vi "Test DAQmx With Queues.vi"() -> ()   [LabVIEW 2019, in "DAQmx.lvclass"]
uses:
  DAQmx.lvclass
  typedefs/DAQ.Configuration--Cluster.ctl
  typedefs/DAQ.Config.Timing--Cluster.ctl
  typedefs/DAQ.Config.Timing.Sampling--Cluster.ctl
  typedefs/DAQ.Config.Timing.Fs Mode--enum.ctl
  typedefs/DAQ.Config.AO--Cluster--Array.ctl
  typedefs/DAQ.Config.AO--Cluster.ctl
  typedefs/DAQ.Config.AO.Range--enum.ctl
  typedefs/DAQ.Config.Device Type--enum.ctl
  typedefs/DAQ.Config.AI--Cluster--Array.ctl
  typedefs/DAQ.Config.AI--Cluster.ctl
  typedefs/DAQ.Config.AI.Coupling--enum.ctl
  typedefs/DAQ.Config.AI.Range--enum.ctl
  typedefs/DAQ.Calibration--Cluster--Array.ctl
  typedefs/DAQ.Calibration--Cluster.ctl
  DAQmx.lvclass/DAQmx.ctl
panel:
  out "Waveform Chart":i32(graph)
  out "Generator create":i32
  out "Generator 'timeout'":i32
  out "DAQ 'timeout'":i32
  out "Generator":i32
  out "DAQ":i32
  out "Waveform Graph":waveform(dbl)[](graph)
  in  "stop":bool
  in  "Configuration":T1={"Timing"={"Sampling"={"Fs"=52000.0, "#s"=5000}, "sample mode"=10123, "FsMode"=enum."Manual", "Fs Multiplier"=1.0, "Refresh Rate (Hz)"=10.0, "Decimation.PreDSP"=1, "Decimation.PostDSP"=1, "Fs.Output"=204789.0}, "AO"=[{"Channels"="PXI1Slot3/ao0", "Range"=enum."±1.0", "output terminal configuration"=-1, "Type"=enum."None"}, {"Channels"="PXI1Slot3/ao1", "Range"=enum."±1.0", "output terminal configuration"=-1, "Type"=enum."None"}, {"Channels"="PXI1Slot5/ao0", "Range"=enum."±1.0", "output terminal configuration"=-1, "Type"=enum."None"}, {"Channels"="PXI1Slot5/ao1", "Range"=enum."±1.0", "output terminal configuration"=-1, "Type"=enum."None"}], "AI"=[{"Channels"="PXI1Slot3/ai0", "Coupling"=10050, "Range"=enum."±0.316", "input terminal configuration"=-1, "Type"=enum."None"}, {"Channels"="PXI1Slot3/ai1", "Coupling"=10050, "Range"=enum."±0.316", "input terminal configuration"=-1, "Type"=enum."None"}, {"Channels"="PXI1Slot5/ai0", "Coupling"=10050, "Range"=enum."±0.316", "input terminal configuration"=-1, "Type"=enum."None"}, {"Channels"="PXI1Slot5/ai1", "Coupling"=10050, "Range"=enum."±0.316", "input terminal configuration"=-1, "Type"=enum."None"}], "Calibration"=[]} {"Calibration"."DevTemp" format="%.1f"; "Calibration"."SelfCal.LastTemp" format="%.1f"; "Calibration"."SelfCal.LastDate/Time" format="%<%I:%M %p %m/%d/%Y>T"; "AI"."input terminal configuration" items=[""=-1, "Differential"=10106, "Pseudodifferential"=12529]; "AI"."Coupling" items=[""=0, "AC"=10045, "DC"=10050, "GND"=10066]; "AO"."output terminal configuration" items=[""=-1, "Differential"=10106, "Pseudodifferential"=12529]; "Timing"."Sampling"."Fs" format="%#_13g"}
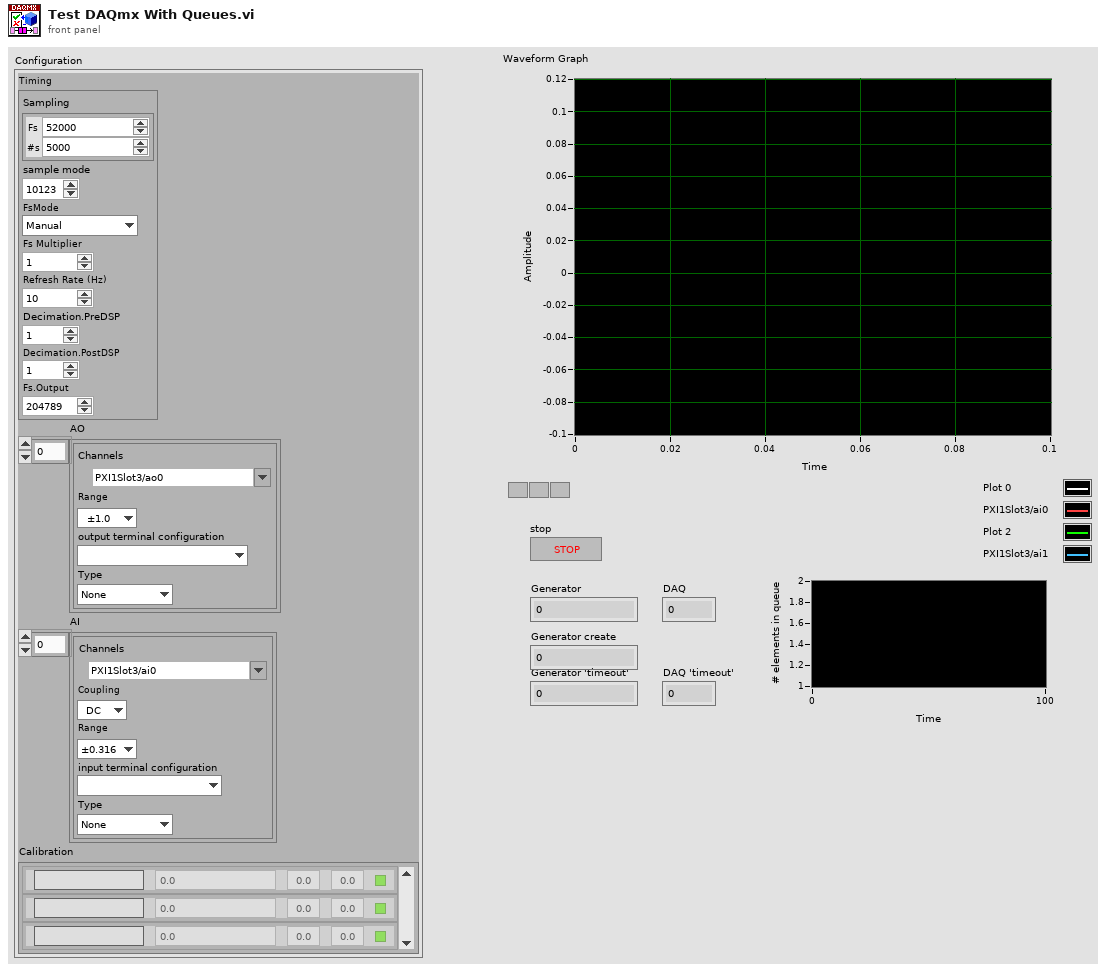
[diagram p1: front panel]
types:
  T1 = typedef "DAQmx.lvclass/DAQ.Configuration--Cluster.ctl" = cluster{"Timing":T2, "AO":T5, "AI":T9, "Calibration":T13}
  T2 = typedef "DAQmx.lvclass/DAQ.Config.Timing--Cluster.ctl" = cluster{"Sampling":T3, "sample mode":i32, "FsMode":T4, "Fs Multiplier":dbl, "Refresh Rate (Hz)":dbl, "Decimation.PreDSP":i32, "Decimation.PostDSP":i32, "Fs.Output":dbl}
  T3 = typedef "DAQmx.lvclass/DAQ.Config.Timing.Sampling--Cluster.ctl" = cluster{"Fs":dbl, "#s":i32}
  T4 = typedef "DAQmx.lvclass/DAQ.Config.Timing.Fs Mode--enum.ctl" = enum16{"Manual", "Auto Fs", "Max Fs"}
  T5 = typedef "DAQmx.lvclass/DAQ.Config.AO--Cluster--Array.ctl" = T6[]
  T6 = typedef "DAQmx.lvclass/DAQ.Config.AO--Cluster.ctl" = cluster{"Channels":tag, "Range":T7, "output terminal configuration":i32, "Type":T8}
  T7 = typedef "DAQmx.lvclass/DAQ.Config.AO.Range--enum.ctl" = enum16{"±0.1", "±1.0", "±10.0", ""}
  T8 = typedef "DAQmx.lvclass/DAQ.Config.Device Type--enum.ctl" = enum16{"None", "USB-4431", "PXI-446x"}
  T9 = typedef "DAQmx.lvclass/DAQ.Config.AI--Cluster--Array.ctl" = T10[]
  T10 = typedef "DAQmx.lvclass/DAQ.Config.AI--Cluster.ctl" = cluster{"Channels":tag, "Coupling":T11, "Range":T12, "input terminal configuration":i32, "Type":T8}
  T11 = typedef "DAQmx.lvclass/DAQ.Config.AI.Coupling--enum.ctl" = u16
  T12 = typedef "DAQmx.lvclass/DAQ.Config.AI.Range--enum.ctl" = enum16{"±0.316", "±1.00", "±3.16", "±10.0", "±31.6", "±42.4", ""}
  T13 = typedef "DAQmx.lvclass/DAQ.Calibration--Cluster--Array.ctl" = T14[]
  T14 = typedef "DAQmx.lvclass/DAQ.Calibration--Cluster.ctl" = cluster{"Active Device":string, "SelfCal.LastDate/Time":dbl, "SelfCal.LastTemp":dbl, "DevTemp":dbl, "calibration due?":bool}
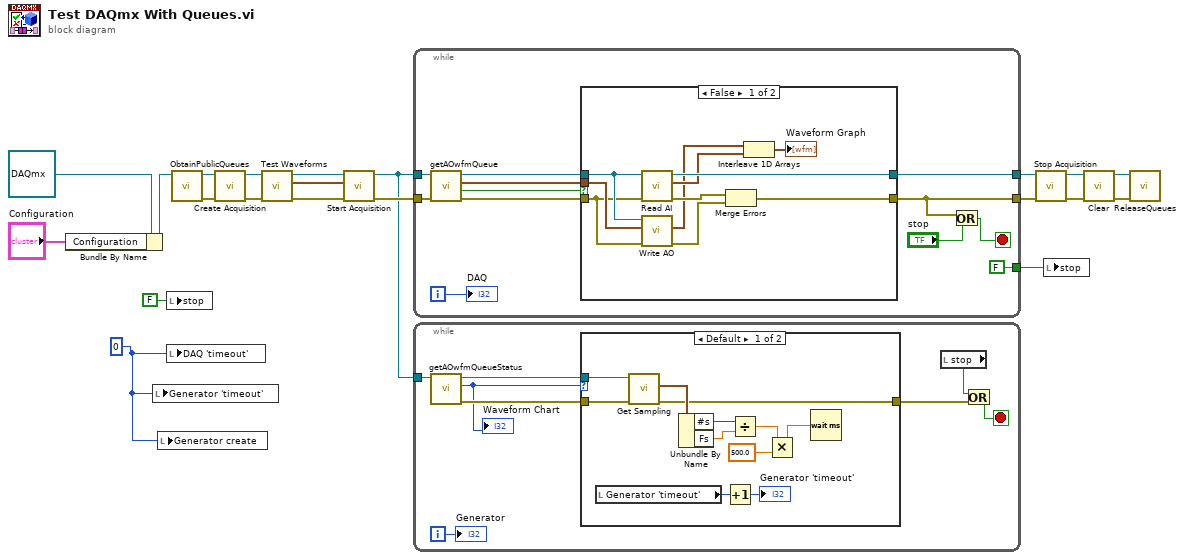
[diagram p0: block diagram]
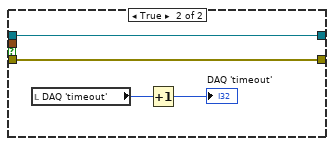
[diagram p2: hidden frame]
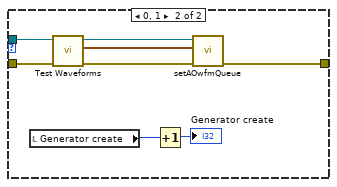
[diagram p3: hidden frame]
diagram:
  w14 = 0 ("consumer 2")
  n1 = Bundle By Name(cluster=refnum<class "DAQmx.lvclass"> refnum ("DAQmx in"), "Configuration"="Configuration") -> (w5:refnum<class "DAQmx.lvclass">)
  n2 = local write "Generator 'timeout'"(w14) -> ()
  n3 = local write "Generator create"(w14) -> ()
  n4 = local write "stop"(FALSE ("stop")) -> ()
  n5 = local write "DAQ 'timeout'"(w14) -> ()
  n6 = call "ObtainPublicQueues.vi"("DAQmx"=w5) -> ("error out"=w4:errorcluster, "DAQmx out"=w6:refnum<class "DAQmx.lvclass">)  [unwired: 9 in]
  n7 = call "Create Acquisition.vi"("error in"=w4, "DAQmx in"=w6) -> ("error out"=w10:errorcluster, "DAQmx out"=w11:refnum<class "DAQmx.lvclass">)  [unwired: 8 in]
  n8 = call "Test Waveforms.vi"("error in (no error)"=w10, "DAQmx in"=w11) -> ("error out"=w1:errorcluster, "Array"=w8:waveform(dbl)[], "DAQmx out"=w9:refnum<class "DAQmx.lvclass">)  [unwired: 7 in]
  n9 = call "Start Acquisition.vi"("error in"=w1, "WFM in"=w8, "DAQmx in"=w9) -> ("error out"=w12:errorcluster, "DAQmx out"=w7:refnum<class "DAQmx.lvclass">)  [unwired: 7 in]
  n10 = while {
    tunnel: w7 -> [w26]
    tunnel: [w33] -> w19
    tunnel: [w29] -> w16
    tunnel: w12 -> [w22]
    tunnel: [FALSE ("stop")] -> w13
    i -> [w30]
    stop <- w31 stop-if-true
    n11 = call "getAOwfmQueue.vi"("error in (no error)"=w22, "DAQmx in"=w26) -> ("error out"=w23:errorcluster, "timed out?"=w24:bool, "AOwfm"=w25:waveform(dbl)[], "DAQmx out"=w27:refnum<class "DAQmx.lvclass">)  [unwired: 6 in]
    n12 = case shown="False" w24 {
      tunnel: [w43 w47] -> w33
      tunnel: [w38 w46] -> w29
      tunnel: w27 -> [w37 w47]
      tunnel: w25 -> [w36 _]
      tunnel: w23 -> [w34 w46]
      frame False {
        n13 = call "Read AI.vi"("error in"=w34, "DAQmx in"=w37) -> ("error out"=w42:errorcluster, "Awfm"=w40:waveform(dbl)[], "DAQmx out"=w43:refnum<class "DAQmx.lvclass">)  [unwired: 6 in, 1 out]
        n14 = call "Write AO.vi"("error in (no error)"=w34, "AOwfm"=w36, "DAQmx in"=w37) -> ("error out"=w39:errorcluster, "AOwfm out (previous)"=w35:waveform(dbl)[])  [unwired: 5 in, 2 out]
        n15 = Merge Errors(w42, w39) -> (w38:errorcluster)
        n16 = Interleave 1D Arrays(w35, w40) -> (→"Waveform Graph":waveform(dbl)[])
      }
      frame True {
        n17 = local read "DAQ 'timeout'"() -> (w45:i32)
        n18 = Increment(x=w45) -> (x+1=→"DAQ 'timeout'":i32)
      }
    }
    n19 = Or(x=w29, y="stop") -> (x .or. y?=w31:bool)
    "DAQ" <- w30
  }
  n20 = while {
    tunnel: w7 -> [w51]
    i -> [w55]
    stop <- w53 stop-if-true
    n21 = call "getAOwfmQueueStatus.vi"("DAQmx in"=w51) -> ("error out"=w50:errorcluster, "# elements in queue"=w48:i32, "DAQmx out"=w52:refnum<class "DAQmx.lvclass">)  [unwired: 8 in]
    "Waveform Chart" <- w48
    n22 = case shown="Default" w48 {
      tunnel: w52 -> [w59 w72]
      tunnel: w50 -> [w58 w69]
      tunnel: [w56 w67] -> w49
      frame Default {
        n23 = local read "Generator 'timeout'"() -> (w66:i32)
        n24 = call "Get Sampling.vi"("error in (no error)"=w58, "DAQmx in"=w59) -> ("error out"=w56:errorcluster, "Sampling info"=w57:T3)  [unwired: 7 in, 1 out]
        n25 = Unbundle By Name(w57) -> ("#s"=w64:i32, "Fs"=w63:dbl)
        n26 = Increment(x=w66) -> (x+1=→"Generator 'timeout'":i32)
        n27 = Divide(x=w64, y=w63) -> (x/y=w61:dbl)
        n28 = Multiply(x=w61, y=500.0) -> (x*y=w60:dbl)
        n29 = Wait (ms)(milliseconds to wait=w60) -> ()  [unwired: 1 out]
      }
      frame 0, 1 {
        n30 = local read "Generator create"() -> (w73:i32)
        n31 = call "Test Waveforms.vi"("error in (no error)"=w69, "DAQmx in"=w72) -> ("error out"=w68:errorcluster, "Array"=w70:waveform(dbl)[], "DAQmx out"=w71:refnum<class "DAQmx.lvclass">)  [unwired: 7 in]
        n32 = Increment(x=w73) -> (x+1=→"Generator create":i32)
        n33 = call "setAOwfmQueue.vi"("error in (no error)"=w68, "AOwfm"=w70, "DAQmx in"=w71) -> ("error out"=w67:errorcluster)  [unwired: 7 in, 1 out]
      }
    }
    n34 = local read "stop"() -> (w54:bool)
    n35 = Or(x=w54, y=w49) -> (x .or. y?=w53:bool)
    "Generator" <- w55
  }
  n36 = call "Stop Acquisition.vi"("error in (no error)"=w16, "DAQmx in"=w19) -> ("error out"=w17:errorcluster, "DAQmx out"=w18:refnum<class "DAQmx.lvclass">)  [unwired: 8 in]
  n37 = local write "stop"(w13) -> ()
  n38 = call "Clear.vi"("error in (no error)"=w17, "DAQmx in"=w18) -> ("error out"=w2:errorcluster, "DAQmx out"=w3:refnum<class "DAQmx.lvclass">)  [unwired: 8 in]
  n39 = call "ReleaseQueues.vi"("error in (no error)"=w2, "DAQmx"=w3) -> ()  [unwired: 8 in, 2 out]
